vi "VertexArray2dTo3d.vi"(10 "Z":dbl, 11 "VertexArray2D":T2[](array[typedef])) -> (3 "VertexArray3D":T1[](array[typedef]))   [LabVIEW 2014]
uses:
  TypeDefs/Point2D.ctl
  TypeDefs/Point3D.ctl
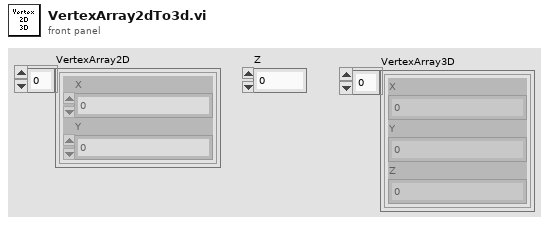
[diagram p1: front panel]
types:
  T1 = typedef "Point3D.ctl" = cluster{"X":sgl, "Y":sgl, "Z":sgl}
  T2 = typedef "Point2D.ctl" = cluster{"X":sgl, "Y":sgl}
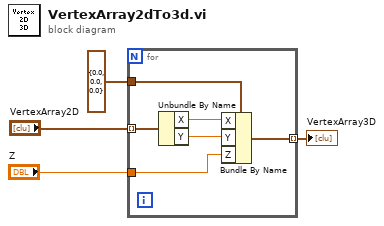
[diagram p0: block diagram]
diagram:
  n1 = for {
    tunnel: "VertexArray2D" -> [w9] mode=indexing
    tunnel: "Z" -> [w8]
    tunnel: T1 {"X"=0.0, "Y"=0.0, "Z"=0.0} ("Point3D") -> [w10]
    tunnel: [w5] -> w1 mode=indexing
    n2 = Unbundle By Name(w9) -> ("X"=w7:sgl, "Y"=w6:sgl)
    n3 = Bundle By Name(cluster=w10, "X"=w7, "Y"=w6, "Z"=w8) -> (w5:T1)
  }
  "VertexArray3D" <- w1
